vi "LitePoint_GPRF_VSA_ReceivedPower.vi"(8 "error in (no error)":errorcluster, 11 "VISA resource name":refnum<visa-resource-name>) -> (0 "error out":errorcluster, 3 "VISA resource name out":refnum<visa-resource-name>, 4 "Power":sgl)   [LabVIEW 2020, in "LitePoints.lvlib"]
uses:
  LitePoints.lvlib
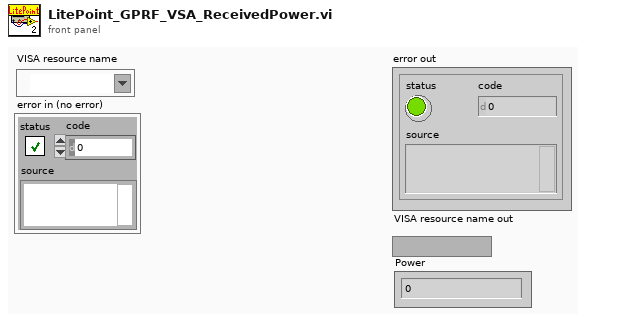
[diagram p1: front panel]
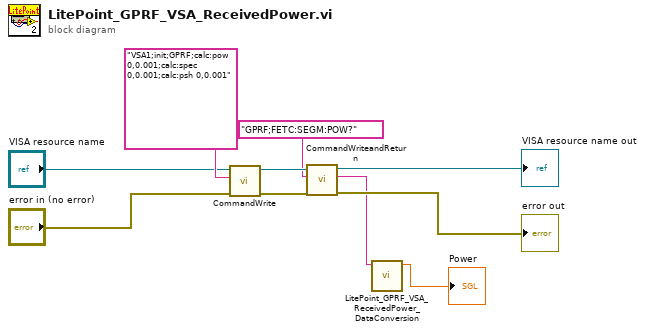
[diagram p0: block diagram]
diagram:
  n1 = call "CommandWrite.vi"("error in (no error)"="error in (no error)", "Write Buffer"="VSA1;init;GPRF;calc:pow 0,0.001;calc:spec 0,0.001;calc:psh 0,0.001", "VISA resource name"="VISA resource name") -> ("error out"=w8:errorcluster, "VISA resource name out"=w9:refnum<visa-resource-name>)  [unwired: 7 in]
  n2 = call "CommandWriteandReturn.vi"("error in (no error)"=w8, "Write Buffer"="GPRF;FETC:SEGM:POW?", "VISA resource name"=w9) -> ("error out"=→"error out":errorcluster, "read buffer"=w2:string, "VISA resource name out"=→"VISA resource name out":refnum<visa-resource-name>)  [unwired: 5 in, 1 out]
  n3 = call "LitePoint_GPRF_VSA_ReceivedPower_DataConversion.vi"("read buffer"=w2) -> ("value"=→"Power":sgl)  [unwired: 10 in]
